vi "Set Output Line.vi"(8 "Error In":errorcluster, 9 "Line":i32, 10 "Value":bool, 11 "BNT_ULx-MCSV in":refnum<class "BNT_ULx-MCSV.lvclass">) -> (0 "Error Out":errorcluster, 3 "BNT_ULx-MCSV out":refnum<class "BNT_ULx-MCSV.lvclass">)   [LabVIEW 2020, in "BNT_ULx.lvlib" / "BNT_ULx-MCSV.lvclass"]
doc: "Write line value to DAQmx device and publish.\n\nTimeout is set to constant 1s."
uses:
  BNT_ULx-MCSV.lvclass
  BNT_ULx-MCSV.lvclass/BNT_ULx-MCSV.ctl
  <vilib>/ULx/Write.llb/ULx Write (Digital 1D Bool NChan 1Samp 1Line).vi
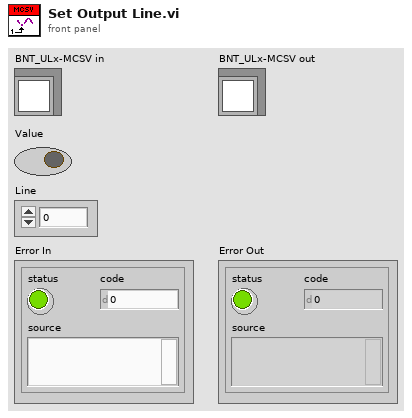
[diagram p1: front panel]
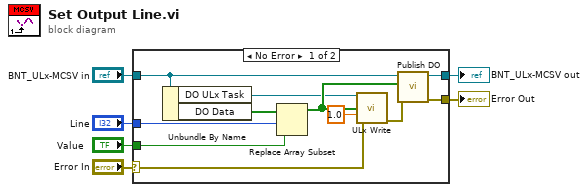
[diagram p0: block diagram]
diagram:
  n1 = case shown="No Error" "Error In" {
    selector: "Error In" -> [w10 w19]
    tunnel: [w13 w19] -> w5
    tunnel: [w12 w18] -> w3
    tunnel: "BNT_ULx-MCSV in" -> [w14 w18]
    tunnel: "Value" -> [w15 _]
    tunnel: "Line" -> [w16 _]
    frame No Error {
      n2 = Unbundle By Name(w14) -> ("DO ULx Task"=w8:refnum<k24>, "DO Data"=w17:bool[])
      n3 = Replace Array Subset(array=w17, new element=w15, index=w16) -> (w11:bool[])
      n4 = call-poly <vilib>:"ULx Write.vi"("task in"=w8, "data"=w11, "timeout"=1.0, "error in"=w10) -> ("error out"=w7:errorcluster)  [unwired: 9 in, 2 out]
      n5 = call "Publish DO.vi"("error in"=w7, "DO Data"=w11, "BNT_ULx-MCSV in"=w14) -> ("error out"=w13:errorcluster, "BNT_ULx-MCSV out"=w12:refnum<class "BNT_ULx-MCSV.lvclass">)  [unwired: 7 in]
    }
    frame Error {
    }
  }
  "Error Out" <- w5
  "BNT_ULx-MCSV out" <- w3
